vi "PFI-28000-Channel_Get Wizard Mode.vi"(8 "error in (no error)":errorcluster, 11 "PFI-28000-Channel in":refnum<class "PFI-28000-Channel.lvclass">) -> (0 "error out":errorcluster, 2 "Wizard Mode":string, 3 "PFI-28000-Channel out":refnum<class "PFI-28000-Channel.lvclass">)   [LabVIEW 2017, in "PFI-28000-Channel.lvclass"]
uses:
  PFI-28000-Channel.lvclass
  Utilities/PFI-28000-Utils.lvlib
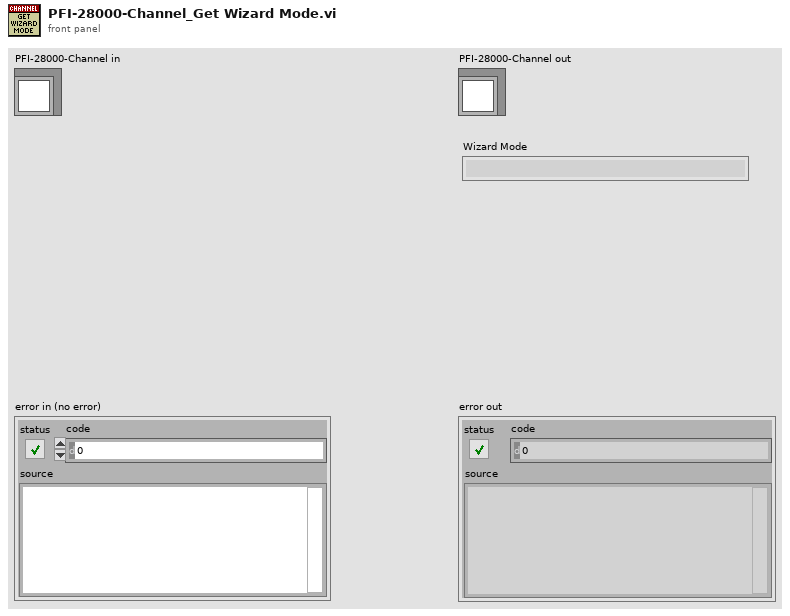
[diagram p1: front panel]
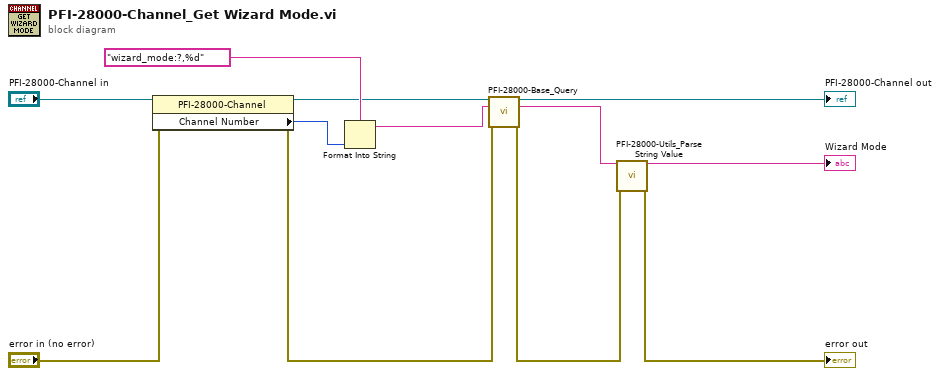
[diagram p0: block diagram]
diagram:
  n1 = property class="PFI-28000-Channel"(reference="PFI-28000-Channel in", error in="error in (no error)") -> (reference out=w6:refnum<class "PFI-28000-Channel.lvclass">, error out=w3:errorcluster, "Channel Number"=w11:i32)
  n2 = Format Into String(format string="wizard_mode:?,%d" ("empty string"), w11) -> (resulting string=w4:string)  [unwired: 2 in, 1 out]
  n3 = call-dynamic "PFI-28000-Base_Query.vi"("PFI-28000-Base in"=w6, "Command"=w4, "error in (no error)"=w3) -> ("PFI-28000-Base out"=→"PFI-28000-Channel out":refnum<class "PFI-28000-Channel.lvclass">, "Response"=w2:string, "error out"=w1:errorcluster)  [unwired: 9 in, 1 out]
  n4 = call "PFI-28000-Utils_Parse String Value.vi"("String"=w2, "error in (no error)"=w1) -> ("String Value"=→"Wizard Mode":string, "error out"=→"error out":errorcluster)  [unwired: 11 in, 1 out]
